vi "_065.vi"() -> ()   [LabVIEW 2024]
uses:
  <vilib>/Utility/inputDevices.llb/keyboardAcquire.vi
  <vilib>/Utility/inputDevices.llb/closeKeyboard.vi
panel:
  in  "stop":bool
  out "keys pressed":T1(array[ring])
  # "Keyboard Control :"
  # "( Using LabVIEW )"
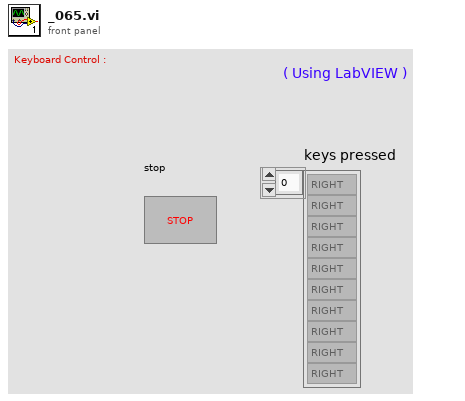
[diagram p1: front panel]
types:
  T1 = enum16{"0", "1", "2", "3", "4", "5", "6", "7", "8", "9", "A", "B", "C", "D", "E", "F", "G", "H", "I", "J", "K", "L", "M", "N", "O", "P", "Q", "R", "S", "T", "U", "V", "W", "X", "Y", "Z", "F1", "F2", "F3", "F4", "F5", "F6", "F7", "F8", "F9", "F10", "F11", "F12", "F13", "F14", "F15", "ADD", "BACK", "BACKSLASH", "CAPITAL", "COMMA", "DECIMAL", "DELETE", "DIVIDE", "DOWN", "END", "EQUALS", "ESCAPE", "GRAVE (`)", "HOME", "INSERT", "LBRACKET", "LCONTROL", "LEFT", "L ALT", "LSHIFT", "LWIN", "MINUS", "MULTIPLY", "NEXT", "NUMLOCK", "NUMPAD_0", "NUMPAD_1", "NUMPAD_2", "NUMPAD_3", "NUMPAD_4", "NUMPAD_5", "NUMPAD_6", "NUMPAD_7", "NUMPAD_8", "NUMPAD_9", "PAUSE", "PERIOD", "PRIOR (PG UP)", "RBRACKET", "RCONTROL", "RETURN", "RIGHT", "R ALT", "RSHIFT", "RWIN", "SCROLL", "SEMICOLON", "SLASH", "SPACE", "SUBTRACT", "TAB", "UP", "ENTER (num pad)", "' (quote)"}[]
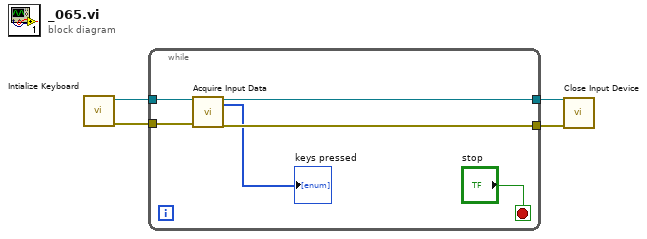
[diagram p0: block diagram]
diagram:
  n1 = call <vilib>:"Intialize Keyboard.vi"() -> ("error out"=w3:errorcluster, "device ID"=w4:refnum<k1>)  [unwired: 10 in]
  n2 = while {
    tunnel: w4 -> [w10]
    tunnel: w3 -> [w9]
    tunnel: [w8] -> w2
    tunnel: [w7] -> w1
    stop <- "stop" stop-if-true
    n3 = call-poly <vilib>:"Acquire Input Data.vi"("device ID"=w10, "error in (no error)"=w9) -> ("device ID"=w8:refnum<k1>, "keys pressed"=→"keys pressed":T1, "error out"=w7:errorcluster)  [unwired: 15 in]
  }
  n4 = call-poly <vilib>:"Close Input Device.vi"("error in (no error)"=w1, "device ID"=w2) -> ()  [unwired: 8 in, 1 out]
